vi "Split.vi"(7 "Average Splitter?":bool, 8 "error in":errorcluster caption="错误输入（无错误）", 10 "Data":variant, 11 "PanelRootNode 输入":refnum<class "PanelRootNode.lvclass"> caption="DNL_LabVIEW Object in") -> (0 "error out":errorcluster caption="错误输出", 3 "PanelRootNode 输出":refnum<class "PanelRootNode.lvclass"> caption="DNL_LabVIEW Object out")   [LabVIEW 2016, in "PanelRootNode.lvclass"]
doc: "本VI作用为分割目标窗格。\n变体Data为含有两个元素的簇，簇中第二个元素为分割模式（横向、纵向等），\n第一个元素可有三种形式：\n1.Node*\n2.Panel Number\n3.Node Path"
uses:
  PanelRootNode.lvclass
  PanelObject/PanelObject.lvclass
  PanelDataNode/Split Mode.ctl
  PanelDataNode/PanelDataNode.lvclass
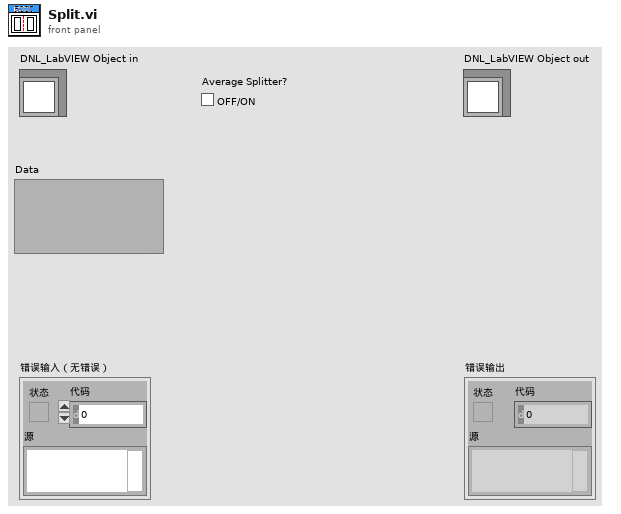
[diagram p1: front panel]
types:
  T1 = typedef "PanelDataNode.lvclass/Split Mode.ctl" = enum16{"Horizontal(up)", "Vertical(left)", "Horizontal(down)", "Vertical(right)"}
  T2 = cluster{"Node*":refnum<data-value>, "Split Mode":T1}
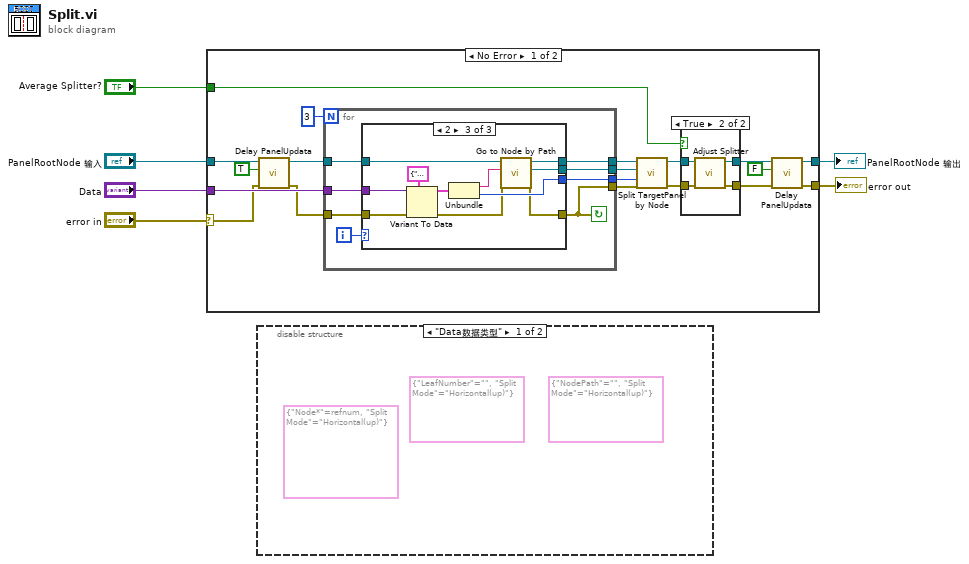
[diagram p0: block diagram]
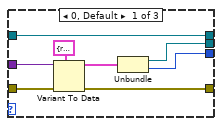
[diagram p4: hidden frame]
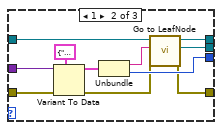
[diagram p5: hidden frame]
diagram:
  n1 = case shown="No Error" "error in" {
    selector: "error in" -> [w17 w71]
    tunnel: [w13 w71] -> w5
    tunnel: [w14 w70] -> w3
    tunnel: "PanelRootNode 输入" -> [w19 w70]
    tunnel: "Data" -> [w20 _]
    tunnel: "Average Splitter?" -> [w7 _]
    frame No Error {
      n2 = call "Delay PanelUpdata.vi"("error in"=w17, "延迟前面板更新"=TRUE, "PanelRootNode 输入"=w19) -> ("error out"=w16:errorcluster, "PanelRootNode 输出"=w18:refnum<class "PanelRootNode.lvclass">)  [unwired: 7 in]
      n3 = for {
        N: 3 -> [_]
        tunnel: [w38] -> w24
        tunnel: [w37] -> w23
        tunnel: w18 -> [w36]
        tunnel: [w35] -> w22
        tunnel: [w34] -> w21
        tunnel: w20 -> [w33]
        tunnel: w16 -> [w32]
        i -> [w39]
        stop <- w34 continue-if-true
        n4 = case shown="2" w39 {
          tunnel: [w47 w58 w69] -> w35
          tunnel: [w46 w53 w64] -> w37
          tunnel: [w42 w56 w66] -> w38
          tunnel: [w43 w52 w63] -> w34
          tunnel: w36 -> [w42 w50 w62]
          tunnel: w33 -> [w41 w49 w60]
          tunnel: w32 -> [w40 w48 w59]
          frame 0, Default {
            n5 = Variant To Data(error in=w40, type=T2 {"Node*"=refnum, "Split Mode"=enum."Horizontal(up)"}, Variant=w41) -> (data=w45:T2, error out=w43:errorcluster)
            n6 = Unbundle(w45) -> ("Node*"=w46:refnum<data-value>, "Split Mode"=w47:T1)
          }
          frame 1 {
            n7 = Variant To Data(error in=w48, type=cluster{string, "Split Mode":T1} {"", "Split Mode"=enum."Horizontal(up)"}, Variant=w49) -> (data=w57:cluster{string, "Split Mode":T1}, error out=w51:errorcluster)
            n8 = Unbundle(w57) -> (w54:string, "Split Mode"=w58:T1)
            n9 = call-dynamic "Go to LeafNode.vi"("error in"=w51, "LeafNumber"=w54, "PanelRootNode 输入"=w50) -> ("error out"=w52:errorcluster, "Node*"=w53:refnum<data-value>, "PanelRootNode 输出"=w56:refnum<class "PanelRootNode.lvclass">)  [unwired: 5 in, 1 out]
          }
          frame 2 {
            n10 = Variant To Data(error in=w59, type=cluster{string, "Split Mode":T1} {"", "Split Mode"=enum."Horizontal(up)"}, Variant=w60) -> (data=w68:cluster{string, "Split Mode":T1}, error out=w61:errorcluster)
            n11 = Unbundle(w68) -> (w65:string, "Split Mode"=w69:T1)
            n12 = call-dynamic "Go to Node by Path.vi"("error in"=w61, "NodePath"=w65, "PanelLinkNode 输入"=w62) -> ("error out"=w63:errorcluster, "Node*"=w64:refnum<data-value>, "PanelLinkNode 输出"=w66:refnum<class "PanelRootNode.lvclass">)  [unwired: 5 in, 1 out]
          }
        }
      }
      n13 = call-dynamic "Split TargetPanel by Node.vi"("error in"=w21, "Split Mode"=w22, "Node*"=w23, "PanelRootNode 输入"=w24) -> ("error out"=w9:errorcluster, "PanelRootNode 输出"=w11:refnum<class "PanelRootNode.lvclass">)  [unwired: 5 in, 1 out]
      n14 = case shown="True" w7 {
        tunnel: w11 -> [w27 w31]
        tunnel: [w27 w30] -> w10
        tunnel: w9 -> [w26 w29]
        tunnel: [w26 w28] -> w8
        frame False {
        }
        frame True {
          n15 = call "Adjust Splitter.vi"("error in (no error)"=w29, "PanelRootNode 输入"=w31) -> ("error out"=w28:errorcluster, "PanelRootNode 输出"=w30:refnum<class "PanelRootNode.lvclass">)  [unwired: 8 in]
        }
      }
      n16 = call "Delay PanelUpdata.vi"("error in"=w8, "延迟前面板更新"=FALSE, "PanelRootNode 输入"=w10) -> ("error out"=w13:errorcluster, "PanelRootNode 输出"=w14:refnum<class "PanelRootNode.lvclass">)  [unwired: 7 in]
    }
    frame Error {
    }
  }
  "error out" <- w5
  "PanelRootNode 输出" <- w3
  n17 = disable-structure shown="\"Data数据类型\"" {
    frame condition #0 {
      (unwired) cluster{"NodePath":string, "Split Mode":T1} {"NodePath"="", "Split Mode"=enum."Horizontal(up)"}
      (unwired) cluster{"LeafNumber":string, "Split Mode":T1} {"LeafNumber"="", "Split Mode"=enum."Horizontal(up)"}
      (unwired) T2 {"Node*"=refnum, "Split Mode"=enum."Horizontal(up)"}
    }
    frame condition #1 (active) {
    }
  }
